vi "Color2RGB.vi"(11 "Image Pixels (U32)":u32[][](array[numeric])) -> (1 "Array 3":u8[][](array[numeric]), 2 "Array":u8[][](array[numeric]), 3 "Array 2":u8[][](array[numeric]))   [LabVIEW 2017, in "ImageAcquisitionLibrary.lvlib"]
uses:
  ImageAcquisitionLibrary.lvlib
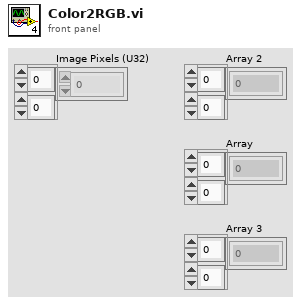
[diagram p1: front panel]
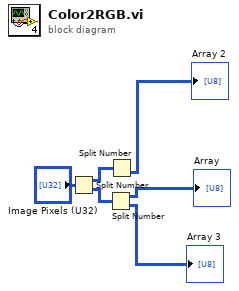
[diagram p0: block diagram]
diagram:
  n1 = Split Number(x="Image Pixels (U32)") -> (hi(x)=w1:u16[][], lo(x)=w2:u16[][])
  n2 = Split Number(x=w2) -> (hi(x)=→"Array":u8[][], lo(x)=→"Array 3":u8[][])
  n3 = Split Number(x=w1) -> (lo(x)=→"Array 2":u8[][])  [unwired: 1 out]
